vi "DynamixelTestForCycleChange.vi"(10 "New position (deg)":dbl, 11 "Old position (deg)":dbl) -> (3 "Dynamixel Cycle Number":i32)   [LabVIEW 2013]
doc: "This VI looks at a Dynamixel position and decides whether it has crossed a boundary line (from 360 to 0 or vice versa) and decides whether the motor cycle should be changed. If the motor has crossed the upper bound of the range the cycle should be incremented, and vice versa.\n\nThis VI assumes that the Dynamixel position is being read often enough to keep the change in position less than 90 degrees from one read to the next.\n\nEric Schneider, April 2014"
panel:
  out "Subtracted value":dbl
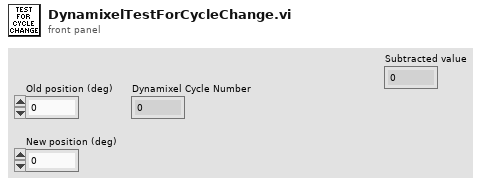
[diagram p1: front panel]
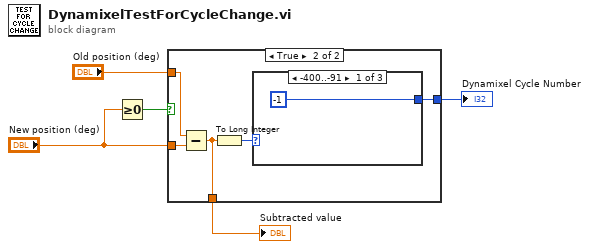
[diagram p0: block diagram]
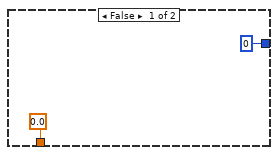
[diagram p2: hidden frame]
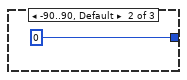
[diagram p3: hidden frame]
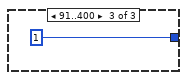
[diagram p4: hidden frame]
diagram:
  n1 = Greater Or Equal To 0?(x="New position (deg)") -> (x >= 0?=w4:bool)
  n2 = case shown="True" w4 {
    tunnel: [0 ("Dynamixel Cycle Number") w11] -> w5
    tunnel: [0.0 w10] -> w3
    tunnel: "Old position (deg)" -> [_ w9]
    tunnel: "New position (deg)" -> [_ w8]
    frame False {
    }
    frame True {
      n3 = Subtract(x=w9, y=w8) -> (x-y=w10:dbl)
      n4 = To Long Integer(number=w10) -> (32bit integer=w12:i32)
      n5 = case shown="-400..-91" w12 {
        tunnel: [-1 ("Dynamixel Cycle Number") 0 ("Dynamixel Cycle Number") 1 ("Dynamixel Cycle Number")] -> w11
        frame -400..-91 {
        }
        frame -90..90, Default {
        }
        frame 91..400 {
        }
      }
    }
  }
  "Dynamixel Cycle Number" <- w5
  "Subtracted value" <- w3
